vi "Calibration_Folder.vi"(11 "input cluster":T1={"L16 Linear Actuator"="", "XE 1000 Pump"="", "Camera1"="", "Camera2"="", "Camera1_IMG"=refnum, "Camera2_IMG"=refnum, "Img_Capt"=FALSE, "Actuator"=FALSE, "Pump"=FALSE, "Cam 1"=FALSE, "Cam 2"=FALSE, "Empty_Refill"=FALSE, "Crop"=FALSE, "Light intensity"=100, "Exposure Time"=1000.0, "Sample Name"="Test Sample", "Operator"="MRJ", "Calibration 1"=path "C:/Users/au540322/Desktop/IHS_Project/images/Debris/Debris_0/Debris_0_2019_06_01-23-32-49-686.PNG", "Calibration 2"=path "C:/Users/au540322/Desktop/IHS_Project/images/Debris/Debris_0/Debris_0_2019_06_01-23-32-49-686.PNG", "Framerate"=1, "Timeout Sample"=50, "Collection date"="MRJ", "Cam 1 queue"=refnum, "Cam 2 queue"=refnum, "Sample size threshold"=1, "Empty start"=1, "Command"="MRJ", "Calibration Image 1"=refnum, "Calibration Image 2"=refnum, "Original Image 1"=refnum, "Original Image 2"=refnum, "Processing Image 1"=refnum, "Processing Image 2"=refnum, "Object Image 1"=refnum, "Object Image 2"=refnum, "Cam 1 - save queue"=refnum, "Cam 2 - save queue"=refnum, "Station"="", "Species Name"="", "Other Notes"="", "Aperture"=enum."Item 0", "Image Process Queue Size"=1, "Image Save Queue Size"=500, "Overload threshold"=500, "Max Framerate"=100, "Blue Plane Image"=refnum, "Subtract Image"=refnum, "Binary Image"=refnum} {"Max Framerate" min=1; "Overload threshold" min=1; "Image Save Queue Size" min=1; "Image Process Queue Size" min=1; "Empty start" min=1; "Sample size threshold" min=1; "Framerate" min=1; "Light intensity" scale=0.0..100.0}) -> (2 "Subfolder Name":string, 3 "Subfolder Path":string)   [LabVIEW 2019]
doc: "Creates folder for storing calibration data and sample configuration setup for further use."
uses:
  controls/Data.ctl
  <vilib>/userdefined/High Color/IMAQdx.ctl
  <vilib>/vision/Image Controls.llb/IMAQ Image.ctl
panel:
  out "error out 2":errorcluster
  out "error out":errorcluster
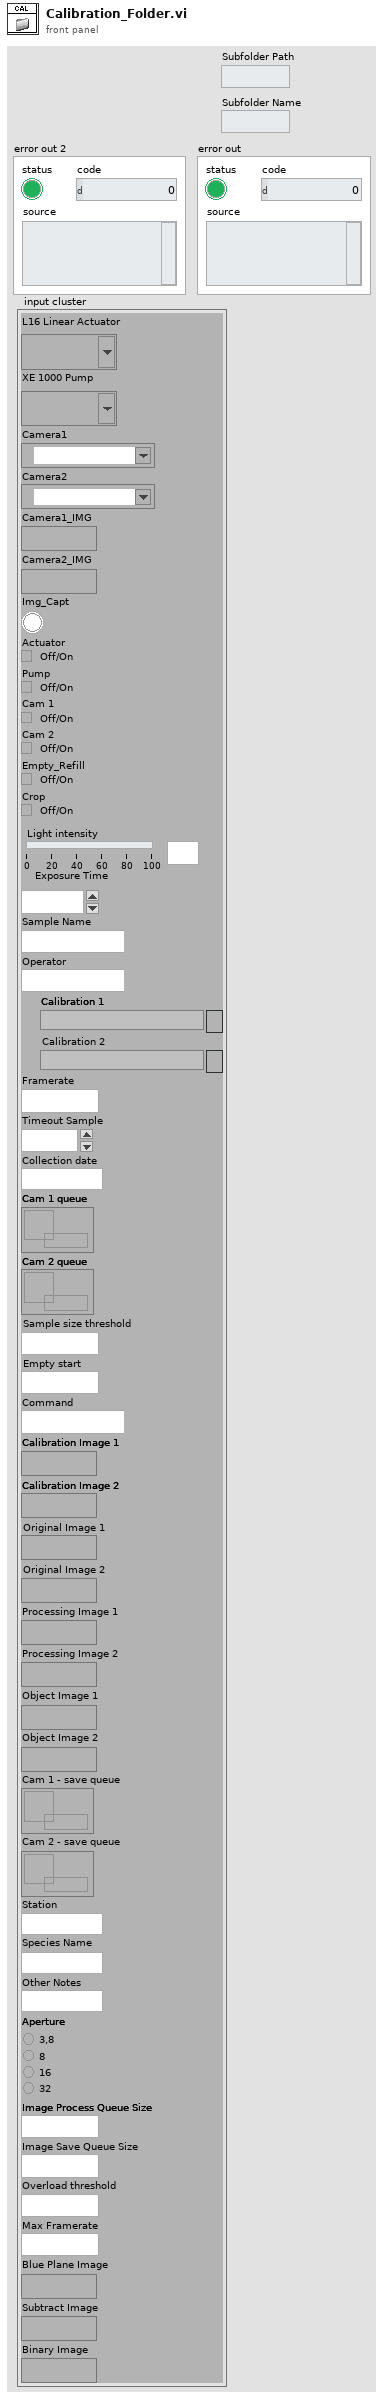
[diagram p1: front panel]
types:
  T1 = typedef "Data.ctl" = cluster{"L16 Linear Actuator":refnum<visa-resource-name>, "XE 1000 Pump":refnum<visa-resource-name>, "Camera1":T2, "Camera2":T2, "Camera1_IMG":T3, "Camera2_IMG":T3, "Img_Capt":bool, "Actuator":bool, "Pump":bool, "Cam 1":bool, "Cam 2":bool, "Empty_Refill":bool, "Crop":bool, "Light intensity":i32, "Exposure Time":dbl, "Sample Name":string, "Operator":string, "Calibration 1":path, "Calibration 2":path, "Framerate":i32, "Timeout Sample":i32, "Collection date":string, "Cam 1 queue":refnum<queue>, "Cam 2 queue":refnum<queue>, "Sample size threshold":i32, "Empty start":u32, "Command":string, "Calibration Image 1":T3, "Calibration Image 2":T3, "Original Image 1":T3, "Original Image 2":T3, "Processing Image 1":T3, "Processing Image 2":T3, "Object Image 1":T3, "Object Image 2":T3, "Cam 1 - save queue":refnum<queue>, "Cam 2 - save queue":refnum<queue>, "Station":string, "Species Name":string, "Other Notes":string, "Aperture":enum32{"Item 0", "Item 1", "Item 2", "Item 3"}, "Image Process Queue Size":i32, "Image Save Queue Size":i32, "Overload threshold":i32, "Max Framerate":i32, "Blue Plane Image":T3, "Subtract Image":T3, "Binary Image":T3}
  T2 = typedef "IMAQdx.ctl" = refnum<k21>
  T3 = typedef "IMAQ Image.ctl" = refnum<image>
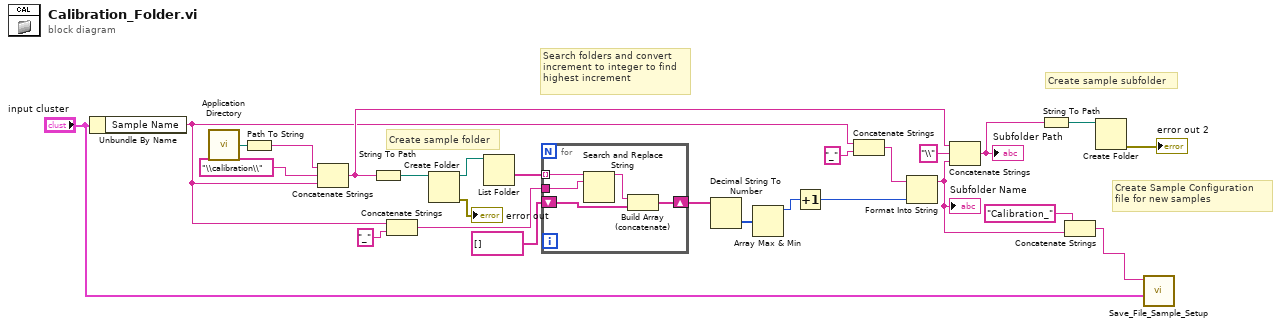
[diagram p0: block diagram]
diagram:
  # "Create Sample Configuration \nfile for new samples"
  # "Create sample subfolder"
  # "Search folders and convert \nincrement to integer to find\nhighest increment"
  # "Create sample folder"
  n1 = Unbundle By Name("input cluster") -> ("Sample Name"=w8:string)
  n2 = call <vilib>:"Application Directory.vi"() -> ("Application Directory"=w18:path)
  n3 = Path To String(path=w18) -> (string=w19:string)
  n4 = Concatenate Strings(w19, "\\calibration\\" ("string"), w8) -> (w10:string)
  n5 = String To Path(string=w10) -> (path=w21:path)
  n6 = Concatenate Strings(w8, "_" ("string")) -> (w16:string)
  n7 = Create Folder(path (use dialog)=w21) -> (created path=w24:path, error out=→"error out":errorcluster)  [unwired: 2 in, 1 out]
  n8 = List Folder(path=w24) -> (folder names=w17:string[])  [unwired: 3 in, 3 out]
  n9 = for {
    tunnel: w17 -> [w31] mode=indexing
    tunnel: w16 -> [w30]
    shift-right: [w28] -> w14
    shift-left: string[] [] -> [w27]
    n10 = Search and Replace String(input string=w31, search string=w30) -> (result string=w29:string)  [unwired: 6 in, 3 out]
    n11 = Build Array (concatenate)(w29, w27) -> (w28:string[])
  }
  n12 = Decimal String To Number(string=w14) -> (number=w13:i32[])  [unwired: 2 in, 1 out]
  n13 = Array Max & Min(array=w13) -> (max value=w12:i32)  [unwired: 3 out]
  n14 = Increment(x=w12) -> (x+1=w1:i32)
  n15 = Concatenate Strings(w8, "_" ("string")) -> (w26:string)
  n16 = Format Into String(initial string=w26, w1) -> (resulting string=w3:string)  [unwired: 2 in, 1 out]
  "Subfolder Name" <- w3
  n17 = Concatenate Strings(w10, "\\" ("string"), w3) -> (w7:string)
  "Subfolder Path" <- w7
  n18 = String To Path(string=w7) -> (path=w9:path)
  n19 = Concatenate Strings("Calibration_" ("string"), w3) -> (w2:string)
  n20 = Create Folder(path (use dialog)=w9) -> (error out=→"error out 2":errorcluster)  [unwired: 2 in, 2 out]
  n21 = call "Save_File_Sample_Setup.vi"("input cluster"="input cluster", "Sample Subfolder Name"=w2) -> ()  [unwired: 9 in, 1 out]
